vi "Initialize.vi"(7 "thread ID":i32, 8 "error in":errorcluster, 9 "component name":string, 10 "Plugin Configuration":refnum<class "Plugin Configuration.lvclass">, 11 "RDMA Transceiver in":refnum<class "RDMA Transceiver.lvclass">) -> (0 "error out":errorcluster, 3 "RDMA Transceiver out":refnum<class "RDMA Transceiver.lvclass">)   [LabVIEW 2020, in "RDMA.lvlib" / "RDMA Transceiver.lvclass"]
doc: "Initializes every level of DSF plugin. Most importantly initializes RDMA sessions."
uses:
  RDMA Transceiver.lvclass
  DSF Core.lvlibp/Classes/Configuration/Core/Plugin/Plugin Configuration.lvclass
  DSF Core.lvlibp/Classes/Configuration/Core/Thread/Thread Configuration.lvclass
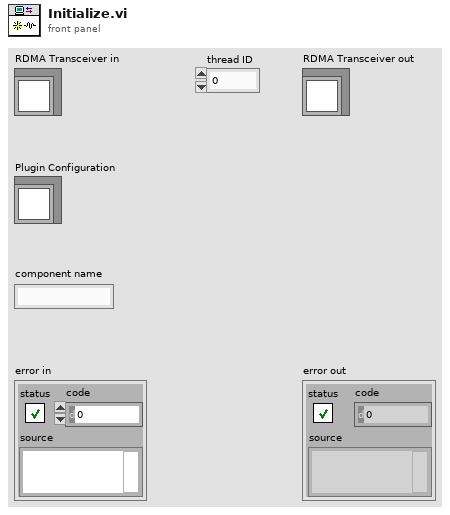
[diagram p1: front panel]
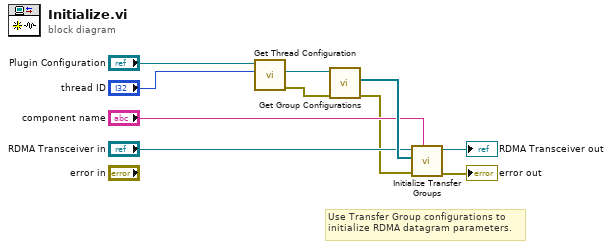
[diagram p0: block diagram]
diagram:
  # "Use Transfer Group configurations to initialize RDMA datagram parameters."
  n1 = call "Get Thread Configuration.vi"("index"="thread ID", "Plugin Configuration in"="Plugin Configuration") -> ("error out"=w2:errorcluster, "Thread Configuration"=w6:refnum<class "Thread Configuration.lvclass">)  [unwired: 7 in, 1 out]
  n2 = call "Get Group Configurations.vi"("error in (no error)"=w2, "Thread Configuration in"=w6) -> ("error out"=w1:errorcluster, "Group Configurations"=w7:refnum<class "Group Configuration.lvclass">[])  [unwired: 7 in, 1 out]
  n3 = call-dynamic "Initialize Transfer Groups.vi"("component name"="component name", "error in"=w1, "Group Configurations"=w7, "RDMA Transceiver in"="RDMA Transceiver in") -> ("error out"=→"error out":errorcluster, "RDMA Transceiver out"=→"RDMA Transceiver out":refnum<class "RDMA Transceiver.lvclass">)  [unwired: 6 in]
